vi "Estructura Evento.vi"() -> ()   [LabVIEW 2020]
panel:
  out "Numeric":i32
  out "NewVal":dbl
  in  "stop":bool
  in  "Slide":dbl(slide) scale=0.0..10.0
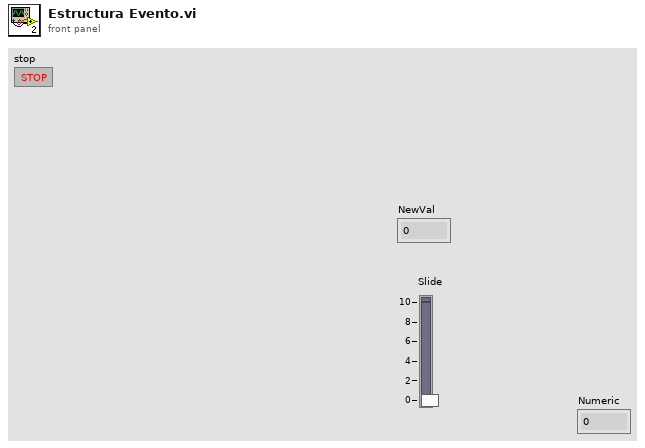
[diagram p1: front panel]
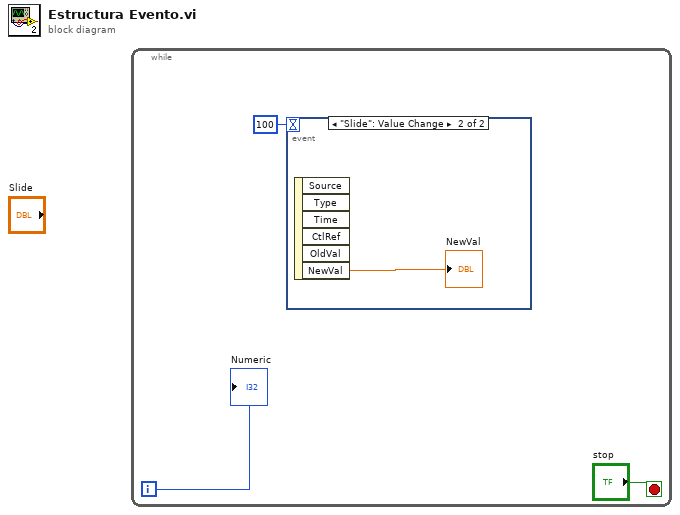
[diagram p0: block diagram]
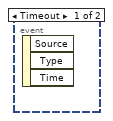
[diagram p2: hidden frame]
diagram:
  n1 = while {
    i -> [w2]
    stop <- "stop" stop-if-true
    n2 = event shown="[1] \"Slide\": Value Change" {
      selector: _ -> [_ _]
      dyn-events: _ -> [_ _]
      timeout: 100 -> [_ _]
      event Timeout {
        n3 = event-data() -> ()  [unwired: 1 in, 3 out]
      }
      event "Slide": Value Change {
        n4 = event-data() -> ("NewVal"=→"NewVal":dbl)  [unwired: 1 in, 5 out]
      }
    }
    "Numeric" <- w2
  }
